vi "Autonomous Independent.vi"() -> ()   [LabVIEW 2017]
doc: "This VI is called when autonomous begins, and will automatically be terminated when autonomous ends. You can carry out timed or sensor driven robot movement independently without needing to return to the caller."
uses:
  <vilib>/Rock Robotics/WPI/ThirdParty/Sensors/navX/_TypeDefs/FRIC_navX_DeviceNumbersTypeDef.ctl
  <vilib>/Rock Robotics/WPI/Utilities/WPI_GetSetVariantRefNum.vi
  <vilib>/Rock Robotics/Network Tables/NT Read String.vi
  <vilib>/Rock Robotics/Network Tables/NT Write Numeric Array.vi
panel:
  out "error out":errorcluster
  out "Array":dbl[](array[numeric])
  out "Direction":string[](array[string])
  # "Be sure to right-click and choose Data Operations>>Make Current Value default if you want to save the array values with the VI"
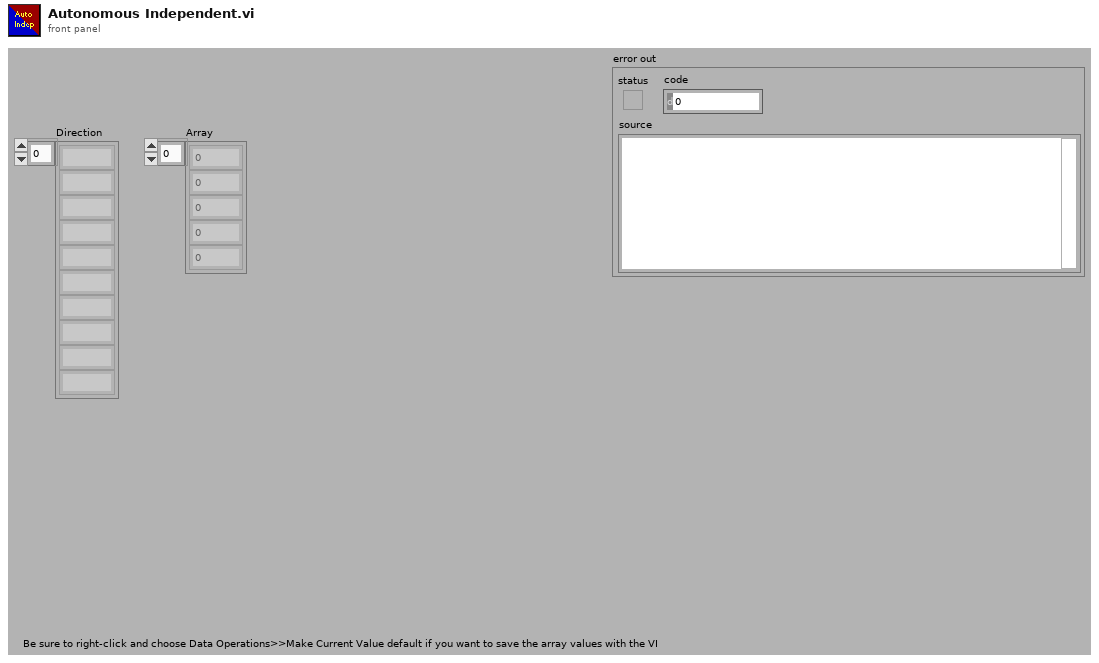
[diagram p1: front panel]
types:
  T1 = typedef "FRIC_navX_DeviceNumbersTypeDef.ctl" = enum16{"Dev0", "Dev1", "Dev2", "Dev3"}
  T2 = cluster{"Left Encoder":string, "Right Encoder":string, "Gyro Refnum":string, "Device Number":T1, "Right Refnum":string, "Left Refnum":string, "Right Intake":string, "Left Intake":string}
  T3 = typedef "WPI_JoystickDevRef.ctl" = cluster{"Device":T4}
  T4 = typedef "WPI_JoystickDeviceEnum.ctl" = enum16{"USB 0", "USB 1", "USB 2", "USB 3", "USB 4", "USB 5"}
  T5 = typedef "WPI_DriverStationPositionInfo.ctl" = enum16{"1", "2", "3"}
  T6 = cluster{"Left Encoder":string, "Right Encoder":string, "Gyro Refnum":string, "Device Number":T1, "Right Refnum":string, "Left Refnum":string, "Left Intake":string, "Right Intake":string}
  T7 = cluster{"Width":u16, "Style":enum32{"Solid", "Dash", "Dot", "DashDot", "DashDotDot"}}
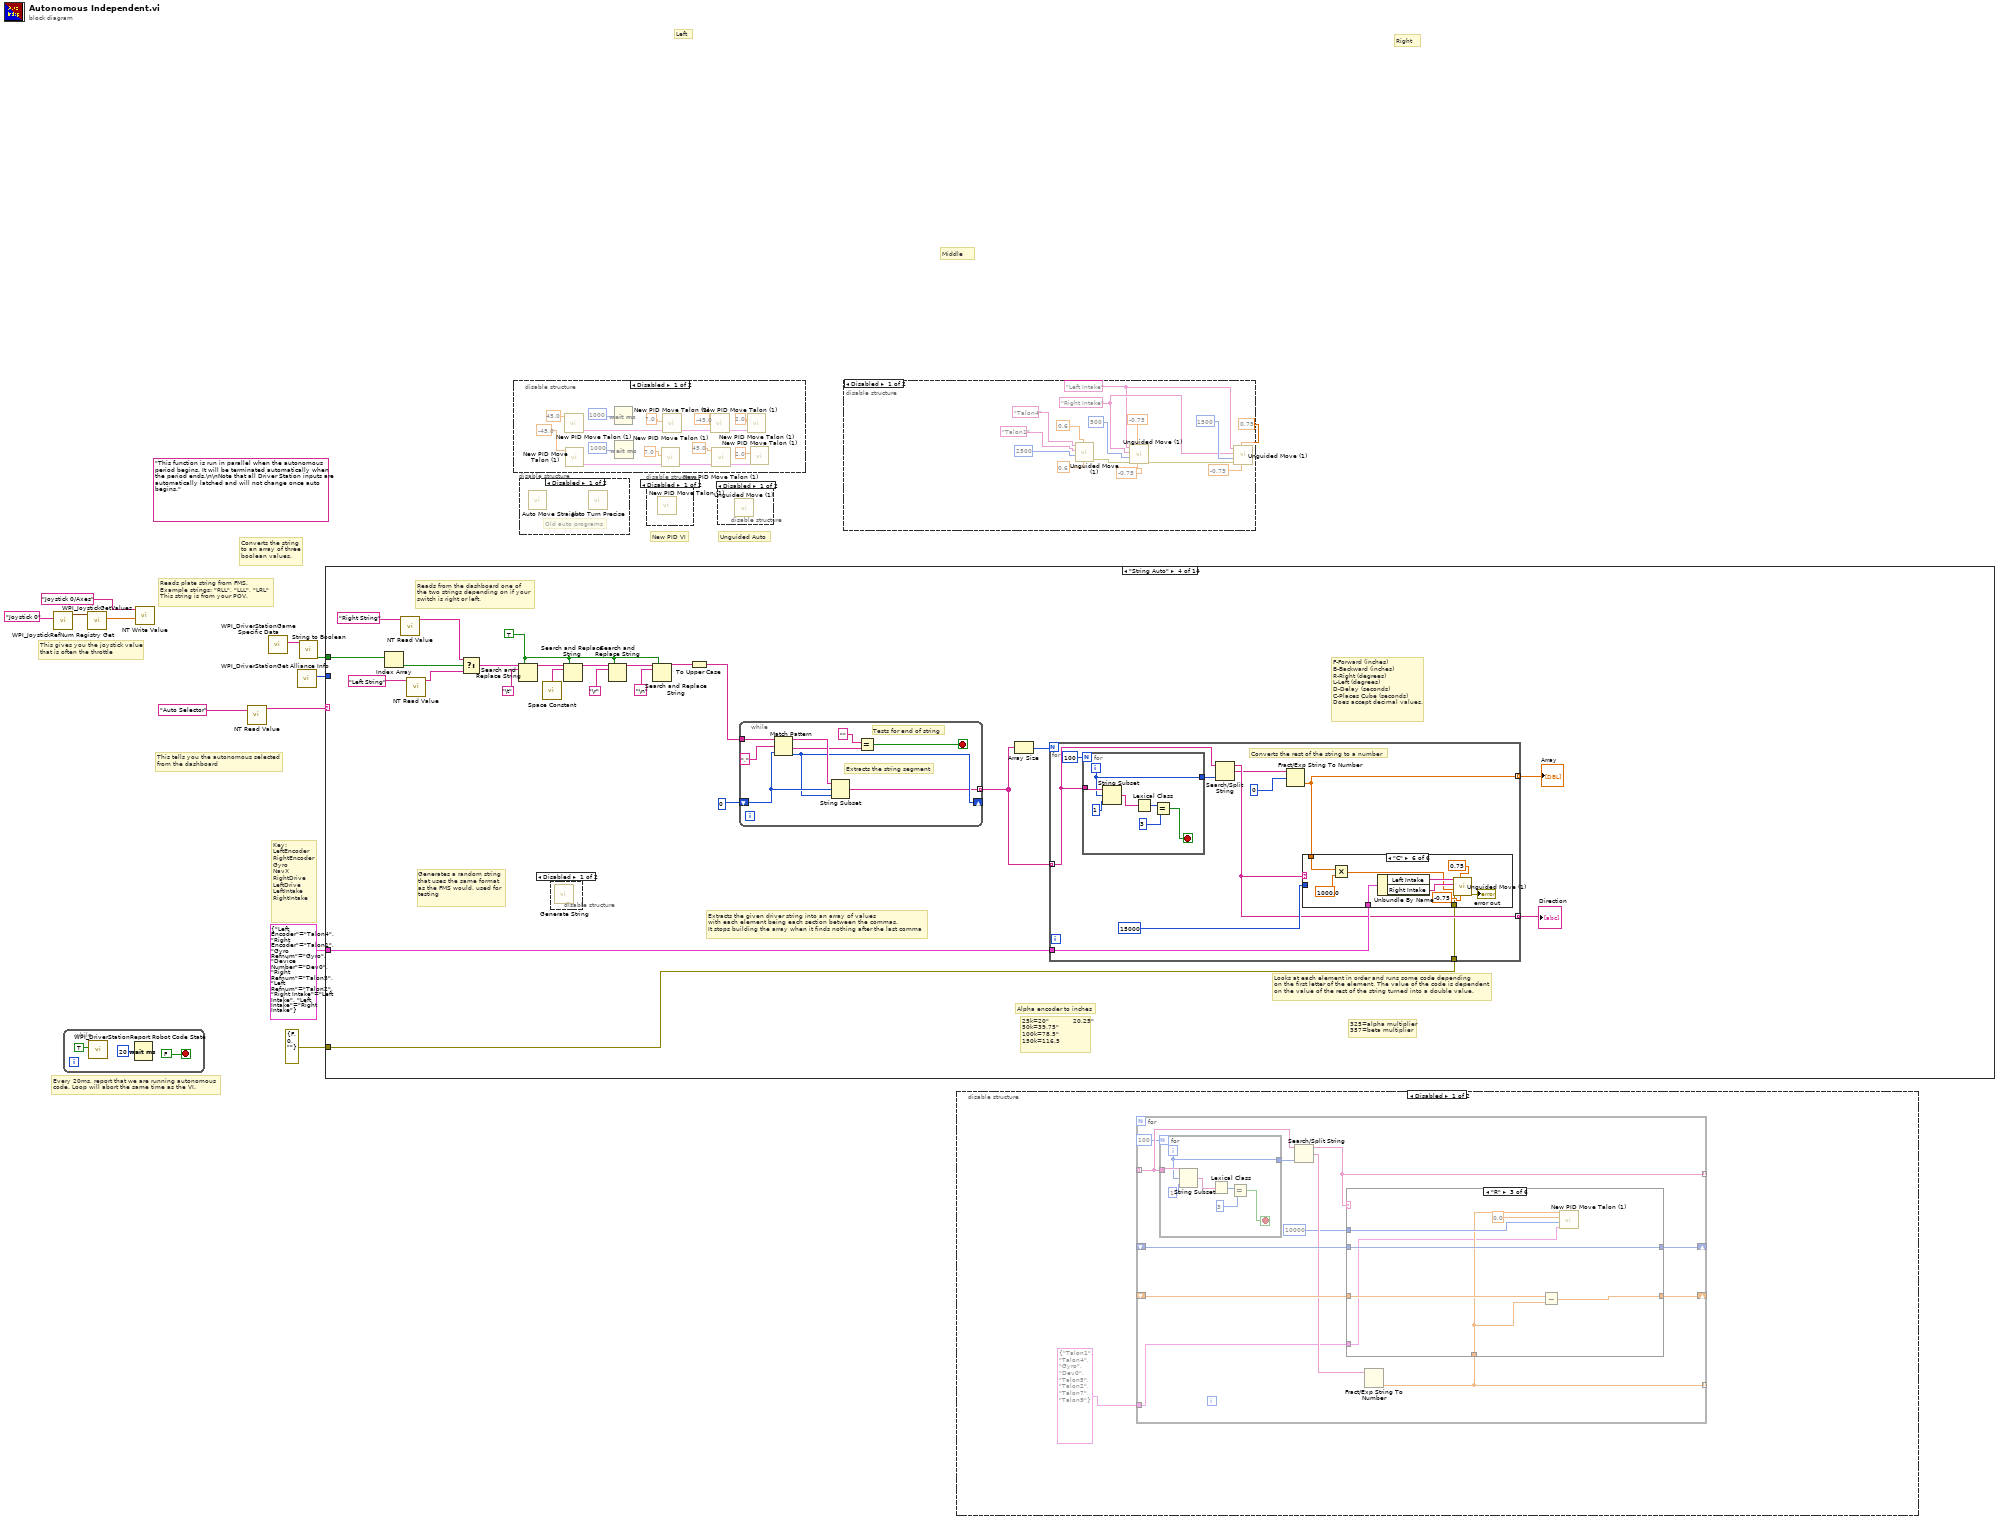
[diagram p0: block diagram]
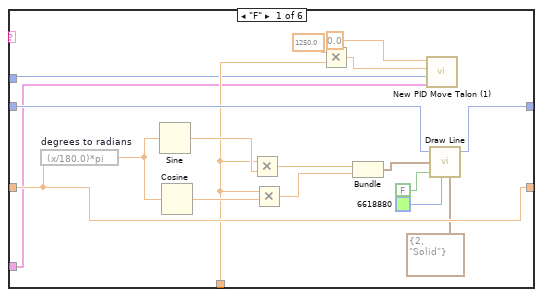
[diagram p2: hidden frame]
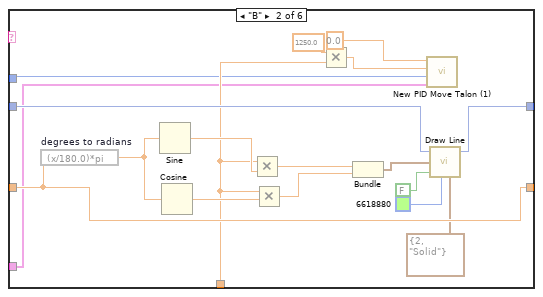
[diagram p3: hidden frame]
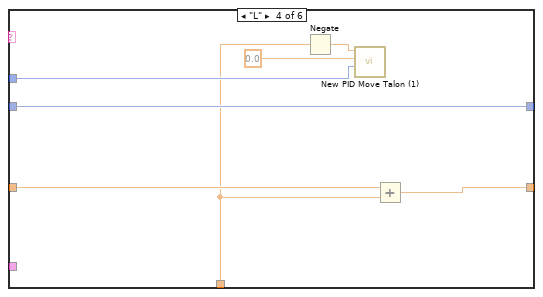
[diagram p4: hidden frame]
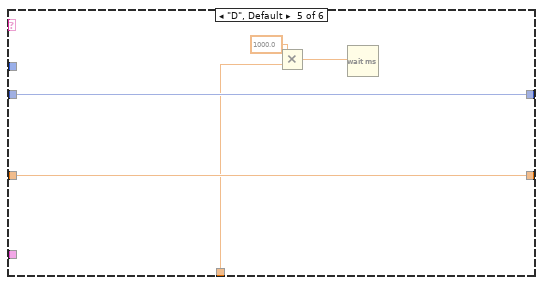
[diagram p5: hidden frame]
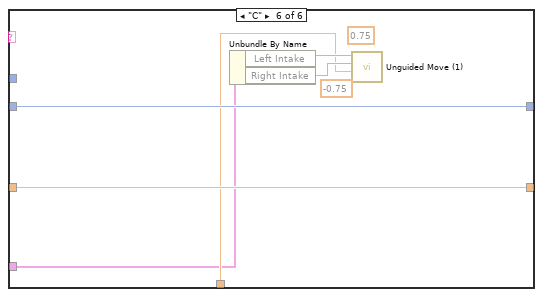
[diagram p6: hidden frame]
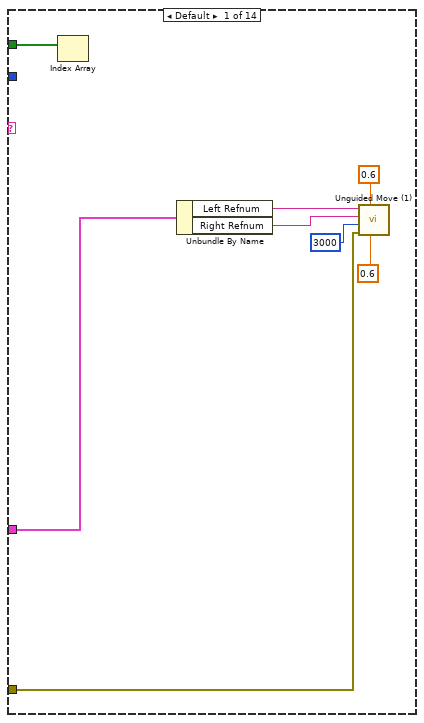
[diagram p13: hidden frame]
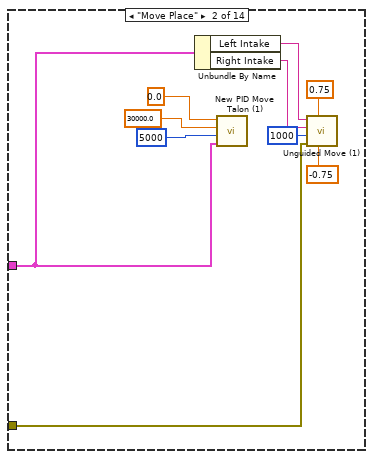
[diagram p14: hidden frame]
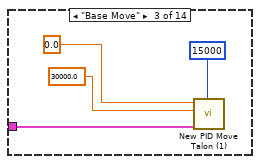
[diagram p15: hidden frame]
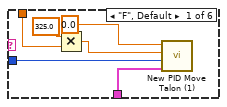
[diagram p17: hidden frame]
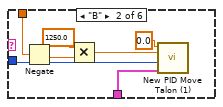
[diagram p18: hidden frame]
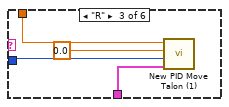
[diagram p19: hidden frame]
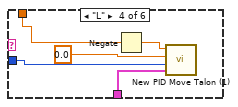
[diagram p20: hidden frame]
diagram:
  (unwired) "This function is run in parallel when the autonomous period begins. It will be terminated automatically when the period ends.\n\nNote that all Driver Station inputs are automatically latched and will not change once auto begins."
  # "Key:\nLeftEncoder\nRightEncoder\nGyro\nNavX\nRightDrive\nLeftDrive\nLeftIntake\nRightIntake"
  # "Unguided Auto"
  # "New PID VI"
  # "Converts the string\nto an array of three\nboolean values."
  # "Reads plate string from FMS. \nExample strings: \"RLL\", \"LLL\", \"LRL\"\nThis string is from your POV."
  # "Middle"
  # "Left"
  # "Right"
  # "This tells you the autonomous selected\nfrom the dashboard"
  # "Every 20ms, report that we are running autonomous\ncode. Loop will abort the same time as the VI."
  # "This gives you the joystick value\nthat is often the throttle"
  n1 = call <vilib>:"WPI_JoystickRefNum Registry Get.vi"("refnum name"="Joystick 0") -> ("JoystickDevRef"=w10:T3)  [unwired: 1 in, 9 out]
  n2 = while {
    stop <- FALSE stop-if-true
    n3 = call <vilib>:"WPI_DriverStationReport Robot Code State.vi"("Autonomous"=TRUE) -> ()  [unwired: 10 in, 1 out]
    n4 = Wait (ms)(milliseconds to wait=u32 20) -> ()  [unwired: 1 out]
  }
  n5 = call <vilib>:"WPI_JoystickGetValues.vi"("JoystickDevRef"=w10) -> ("Axes"=w7:dbl[])  [unwired: 6 in, 4 out]
  n6 = call-poly <vilib>:"NT Write Value.vi"("Numeric Array"=w7, "Name"="Joystick 0/Axes") -> ()  [unwired: 9 in, 1 out]
  n7 = call-poly <vilib>:"NT Read Value.vi"("Name"="Auto Selector") -> ("String"=w8:string)  [unwired: 9 in, 1 out]
  n8 = call <vilib>:"WPI_DriverStationGame Specific Data.vi"() -> ("Game Specific Data"=w5:string)  [unwired: 11 in]
  n9 = call <vilib>:"WPI_DriverStationGet Alliance Info.vi"() -> ("Position"=w1:T5)  [unwired: 6 in, 5 out]
  n10 = call "String to Boolean.vi"("String"=w5) -> ("Boolean Array"=w4:bool[])  [unwired: 10 in]
  n11 = case shown="\"String Auto\"" w8 {
    tunnel: w4 -> [w15 _ _ w50 w124 _ _ w172 _ _ _ _ _ _]
    tunnel: T2 {"Left Encoder"="Talon4", "Right Encoder"="Talon1", "Gyro Refnum"="Gyro", "Device Number"=enum."Dev0", "Right Refnum"="Talon5", "Left Refnum"="Talon2", "Right Intake"="Left Intake", "Left Intake"="Right Intake"} ("Cluster 3") -> [w16 w32 w33 w38 _ _ _ _ _ _ _ _ _ _]
    tunnel: errorcluster {"status"=FALSE, "code"=0, "source"=""} ("error in (no error)") -> [w19 w26 _ w37 _ _ _ _ _ _ _ _ _ _]
    tunnel: w1 -> [_ _ _ _ _ _ _ _ _ _ _ _ _ _]
    frame Default {
      n12 = Index Array(array=w15) -> ()  [unwired: 1 in, 1 out]
      n13 = Unbundle By Name(w16) -> ("Left Refnum"=w22:string, "Right Refnum"=w21:string)
      n14 = call "Unguided Move (1).vi"("Power 2"=0.6, "Power"=0.6, "error in (no error)"=w19, "milliseconds to wait"=u32 3000, "refnum name 2"=w21, "refnum name"=w22) -> ()  [unwired: 5 in, 1 out]
    }
    frame "Move Place" {
      n15 = Unbundle By Name(w32) -> ("Left Intake"=w28:string, "Right Intake"=w27:string)
      n16 = call "New PID Move Talon (1).vi"("Cluster 3"=w32, "Timeout"=i16 5000, "Target Distance"=30000.0, "Target Angle"=0.0) -> ()  [unwired: 7 in, 1 out]
      n17 = call "Unguided Move (1).vi"("Power 2"=-0.75, "Power"=0.75 ("Power 2"), "error in (no error)"=w26, "milliseconds to wait"=u32 1000, "refnum name 2"=w27, "refnum name"=w28) -> ()  [unwired: 5 in, 1 out]
    }
    frame "Base Move" {
      n18 = call "New PID Move Talon (1).vi"("Cluster 3"=w33, "Timeout"=i16 15000, "Target Distance"=30000.0, "Target Angle"=0.0) -> ()  [unwired: 7 in, 1 out]
    }
    frame "String Auto" {
      w42 = TRUE ("replace all? (F)")
      # "325=alpha multiplier\n357=beta multiplier"
      # "F-Forward (inches)\nB-Backward (inches)\nR-Right (degrees)\nL-Left (degrees)\nD-Delay (seconds)\nC-Places Cube (seconds)\nDoes accept decimal values."
      # "Alpha encoder to inches"
      # "25k=20\"            20.25\"\n50k=39.75\"\n100k=78.5\"\n150k=116.5"
      # "Looks at each element in order and runs some code depending\non the first letter of the element. The value of the code is dependent\non the value of the rest of the string turned into a double value."
      # "Extracts the given driver string into an array of values \nwith each element being each section between the commas.\nIt stops building the array when it finds nothing after the last comma"
      # "Reads from the dashboard one of\nthe two strings depending on if your\nswitch is right or left."
      # "Generates a random string\nthat uses the same format \nas the FMS would, used for\ntesting"
      n19 = Index Array(array=w50) -> (element=w60:bool)  [unwired: 1 in]
      n20 = call-poly <vilib>:"NT Read Value.vi"("Name"="Right String") -> ("String"=w59:string)  [unwired: 9 in, 1 out]
      n21 = call-poly <vilib>:"NT Read Value.vi"("Name"="Left String") -> ("String"=w56:string)  [unwired: 9 in, 1 out]
      n22 = Select(t=w59, s=w60, f=w56) -> (s? t:f=w40:string)
      n23 = Search and Replace String(replace all?=w42, input string=w40, search string="\t") -> (result string=w46:string)  [unwired: 5 in, 3 out]
      n24 = call <vilib>:"Space Constant.vi"() -> ("String"=w44:string)
      n25 = disable-structure shown="Disabled" {
        frame Disabled {
          n26 = call "Generate String.vi"() -> ()  [unwired: 11 in, 1 out]
        }
        frame Enabled {
        }
      }
      n27 = Search and Replace String(replace all?=w42, input string=w46, search string=w44) -> (result string=w47:string)  [unwired: 5 in, 3 out]
      n28 = Search and Replace String(replace all?=w42, input string=w47, search string="\r") -> (result string=w48:string)  [unwired: 5 in, 3 out]
      n29 = Search and Replace String(replace all?=w42, input string=w48, search string="\n") -> (result string=w41:string)  [unwired: 5 in, 3 out]
      n30 = To Upper Case(1:w41) -> (0:w39:string)
      n31 = while {
        tunnel: w39 -> [w121]
        shift-right: [w117] -> _
        shift-left: 0 ("offset past match") -> [w118]
        tunnel: [w116] -> w53 mode=indexing
        stop <- w113 stop-if-true
        # "Tests for end of string"
        # "Extracts the string segment"
        n32 = Match Pattern(string=w121, regular expression=",", offset (0)=w118) -> (before substring=w119:string, after substring=w115:string, offset past match=w117:i32)  [unwired: 1 out]
        n33 = String Subset(string=w119, offset (0)=w118, length (rest)=w117) -> (substring=w116:string)
        n34 = Equal?(x="", y=w115) -> (x = y?=w113:bool)
      }
      n35 = Array Size(array=w53) -> (size(s)=w54:i32)
      n36 = for {
        N: w54 -> [_]
        tunnel: w53 -> [w65] mode=indexing
        tunnel: [w69] -> w51 mode=indexing
        tunnel: [w64] -> w52 mode=indexing
        tunnel: w38 -> [w68]
        tunnel: w37 -> [w61]
        # "Converts the rest of the string to a number"
        n37 = for {
          N: 100 -> [_]
          tunnel: w65 -> [w75]
          tunnel: [w72] -> w66
          i -> [w72]
          stop <- w71 stop-if-true
          n38 = String Subset(string=w75, offset (0)=w72, length (rest)=1 ("length (rest)")) -> (substring=w73:string)
          n39 = Lexical Class(1:w73) -> (0:w77:i16)
          n40 = Equal?(x=w77, y=i16 3) -> (x = y?=w71:bool)
        }
        n41 = Search/Split String(string=w65, offset (0)=w66) -> (substring before match=w64:string, match + rest of string=w63:string)  [unwired: 1 in, 1 out]
        n42 = Fract/Exp String To Number(string=w63, offset=0) -> (number=w69:dbl)  [unwired: 2 in, 1 out]
        n43 = case shown="\"C\"" w64 {
          tunnel: w69 -> [w79 w87 w94 w97 w101 w111]
          tunnel: w68 -> [w83 w90 w92 w96 _ w112]
          tunnel: i16 15000 ("Timeout") -> [w82 w89 w91 w95 _ _]
          tunnel: w61 -> [_ _ _ _ _ w103]
          frame "F", Default {
            n44 = Multiply(x=325.0, y=w79) -> (x*y=w78:dbl)
            n45 = call "New PID Move Talon (1).vi"("Cluster 3"=w83, "Timeout"=w82, "Target Distance"=w78, "Target Angle"=0.0) -> ()  [unwired: 7 in, 1 out]
          }
          frame "B" {
            n46 = Negate(x=w87) -> (-x=w86:dbl)
            n47 = Multiply(x=1250.0, y=w86) -> (x*y=w85:dbl)
            n48 = call "New PID Move Talon (1).vi"("Cluster 3"=w90, "Timeout"=w89, "Target Distance"=w85, "Target Angle"=0.0) -> ()  [unwired: 7 in, 1 out]
          }
          frame "R" {
            n49 = call "New PID Move Talon (1).vi"("Cluster 3"=w92, "Timeout"=w91, "Target Distance"=0.0, "Target Angle"=w94) -> ()  [unwired: 7 in, 1 out]
          }
          frame "L" {
            n50 = Negate(x=w97) -> (-x=w98:dbl)
            n51 = call "New PID Move Talon (1).vi"("Cluster 3"=w96, "Timeout"=w95, "Target Distance"=0.0, "Target Angle"=w98) -> ()  [unwired: 7 in, 1 out]
          }
          frame "D" {
            n52 = Multiply(x=1000.0, y=w101) -> (x*y=w100:dbl)
            n53 = Wait (ms)(milliseconds to wait=w100) -> ()  [unwired: 1 out]
          }
          frame "C" {
            n54 = Multiply(x=w111, y=1000.0) -> (x*y=w107:dbl)
            n55 = Unbundle By Name(w112) -> ("Left Intake"=w108:string, "Right Intake"=w109:string)
            n56 = call "Unguided Move (1).vi"("Power 2"=-0.75, "Power"=0.75, "error in (no error)"=w103, "milliseconds to wait"=w107, "refnum name 2"=w109, "refnum name"=w108) -> ("error out"=→"error out":errorcluster)  [unwired: 5 in]
          }
        }
      }
      "Direction" <- w52
      "Array" <- w51
    }
    frame "Front Left Auto" {
      w127 = "Right Intake" ("refnum name")
      w125 = "Left Intake" ("refnum name")
      n57 = Index Array(array=w124) -> (element=w123:bool)  [unwired: 1 in]
      n58 = Not(x=w123) -> (.not. x?=w122:bool)
      n59 = call "Unguided Move (1).vi"("Power 2"=0.6, "Power"=0.6, "milliseconds to wait"=u32 2500, "refnum name 2"="Talon1", "refnum name"="Talon4") -> ("error out"=w129:errorcluster)  [unwired: 6 in]
      n60 = call "Unguided Move (1).vi"("Power 2"=-0.75 ("Power"), "Power"=-0.75, "error in (no error)"=w129, "milliseconds to wait"=u32 500, "refnum name 2"=w127, "refnum name"=w125) -> ("error out"=w126:errorcluster)  [unwired: 5 in]
      n61 = case shown="True" w122 {
        tunnel: w127 -> [_ w142]
        tunnel: w126 -> [_ w139]
        tunnel: w125 -> [_ w138]
        frame False {
        }
        frame True {
          n62 = call "Unguided Move (1).vi"("Power 2"=-0.75, "Power"=0.75, "error in (no error)"=w139, "milliseconds to wait"=u32 1500, "refnum name 2"=w142, "refnum name"=w138) -> ()  [unwired: 5 in, 1 out]
        }
      }
      n63 = disable-structure shown="Enabled" {
        frame Disabled {
          n64 = call "New PID Move Talon (1).vi"("Target Distance"=4.0 ("Target Angle")) -> ("Cluster 2"=w149:T2)  [unwired: 10 in]
          n65 = call "New PID Move Talon (1).vi"("Cluster 3"=w149, "Target Angle"=90.0 ("Target Distance")) -> ("Cluster 2"=w150:T2)  [unwired: 9 in]
          n66 = call "New PID Move Talon (1).vi"("Cluster 3"=w150, "Target Distance"=5.0 ("Target Angle")) -> ("Cluster 2"=w148:T2)  [unwired: 9 in]
          n67 = call "New PID Move Talon (1).vi"("Cluster 3"=w148, "Target Angle"=-90.0 ("Target Distance")) -> ("Cluster 2"=w151:T2)  [unwired: 9 in]
          n68 = call "New PID Move Talon (1).vi"("Cluster 3"=w151, "Target Distance"=5.0) -> ()  [unwired: 9 in, 1 out]
        }
        frame Enabled {
        }
      }
    }
    frame "Side Left Auto" {
      w152 = i16 15000 ("Timeout")
      n69 = call "New PID Move Talon (1).vi"("Timeout"=w152, "Target Distance"=150000.0) -> ("Cluster 2"=w157:T2)  [unwired: 9 in]
      n70 = call "New PID Move Talon (1).vi"("Cluster 3"=w157, "Timeout"=w152, "Target Angle"=90.0) -> ("Cluster 2"=w156:T2)  [unwired: 8 in]
      n71 = call "New PID Move Talon (1).vi"("Cluster 3"=w156, "Timeout"=w152, "Target Distance"=10000.0) -> ()  [unwired: 8 in, 1 out]
    }
    frame "Other Side Left Auto" {
      n72 = call "New PID Move Talon (1).vi"("Target Distance"=18.5 ("Target Angle")) -> ("Cluster 2"=w166:T2)  [unwired: 10 in]
      n73 = call "New PID Move Talon (1).vi"("Cluster 3"=w166, "Target Angle"=90.0 ("Target Distance")) -> ("Cluster 2"=w167:T2)  [unwired: 9 in]
      n74 = call "New PID Move Talon (1).vi"("Cluster 3"=w167, "Target Distance"=18.0 ("Target Angle")) -> ("Cluster 2"=w165:T2)  [unwired: 9 in]
      n75 = call "New PID Move Talon (1).vi"("Cluster 3"=w165, "Target Angle"=90.0 ("Target Distance")) -> ("Cluster 2"=w168:T2)  [unwired: 9 in]
      n76 = call "New PID Move Talon (1).vi"("Cluster 3"=w168, "Target Distance"=5.0) -> ("Cluster 2"=w169:T2)  [unwired: 9 in]
      n77 = call "New PID Move Talon (1).vi"("Cluster 3"=w169, "Target Angle"=90.0) -> ("Cluster 2"=w170:T2)  [unwired: 9 in]
      n78 = call "New PID Move Talon (1).vi"("Cluster 3"=w170, "Target Distance"=1.0) -> ()  [unwired: 9 in, 1 out]
    }
    frame "Front Right Auto" {
      w175 = "Right Intake" ("refnum name")
      w173 = "Left Intake" ("refnum name")
      n79 = Index Array(array=w172) -> (element=w171:bool)  [unwired: 1 in]
      n80 = call "Unguided Move (1).vi"("Power 2"=0.6, "Power"=0.6, "milliseconds to wait"=u32 2500, "refnum name 2"="Talon2", "refnum name"="Talon5") -> ("error out"=w177:errorcluster)  [unwired: 6 in]
      n81 = call "Unguided Move (1).vi"("Power 2"=-0.75 ("Power"), "Power"=-0.75, "error in (no error)"=w177, "milliseconds to wait"=u32 500, "refnum name 2"=w175, "refnum name"=w173) -> ("error out"=w174:errorcluster)  [unwired: 5 in]
      n82 = case shown="True" w171 {
        tunnel: w175 -> [_ w190]
        tunnel: w174 -> [_ w187]
        tunnel: w173 -> [_ w186]
        frame False {
        }
        frame True {
          n83 = call "Unguided Move (1).vi"("Power 2"=-0.75, "Power"=0.75, "error in (no error)"=w187, "milliseconds to wait"=u32 1500, "refnum name 2"=w190, "refnum name"=w186) -> ()  [unwired: 5 in, 1 out]
        }
      }
      n84 = disable-structure shown="Disabled" {
        frame Disabled {
          n85 = call "New PID Move Talon (1).vi"("Target Distance"=4.0 ("Target Angle")) -> ("Cluster 2"=w197:T2)  [unwired: 10 in]
          n86 = call "New PID Move Talon (1).vi"("Cluster 3"=w197, "Target Angle"=-90.0 ("Target Distance")) -> ("Cluster 2"=w198:T2)  [unwired: 9 in]
          n87 = call "New PID Move Talon (1).vi"("Cluster 3"=w198, "Target Distance"=5.0 ("Target Angle")) -> ("Cluster 2"=w196:T2)  [unwired: 9 in]
          n88 = call "New PID Move Talon (1).vi"("Cluster 3"=w196, "Target Angle"=90.0 ("Target Distance")) -> ("Cluster 2"=w199:T2)  [unwired: 9 in]
          n89 = call "New PID Move Talon (1).vi"("Cluster 3"=w199, "Target Distance"=5.0) -> ()  [unwired: 9 in, 1 out]
        }
        frame Enabled {
        }
      }
    }
    frame "Side Right Auto" {
      n90 = call "New PID Move Talon (1).vi"("Target Distance"=12.0) -> ("Cluster 2"=w204:T2)  [unwired: 10 in]
      n91 = call "New PID Move Talon (1).vi"("Cluster 3"=w204, "Target Angle"=-90.0) -> ("Cluster 2"=w203:T2)  [unwired: 9 in]
      n92 = call "New PID Move Talon (1).vi"("Cluster 3"=w203, "Target Distance"=1.5) -> ()  [unwired: 9 in, 1 out]
    }
    frame "Other Side Right Auto" {
      n93 = call "New PID Move Talon (1).vi"("Target Distance"=18.5 ("Target Angle")) -> ("Cluster 2"=w213:T2)  [unwired: 10 in]
      n94 = call "New PID Move Talon (1).vi"("Cluster 3"=w213, "Target Angle"=-90.0 ("Target Distance")) -> ("Cluster 2"=w214:T2)  [unwired: 9 in]
      n95 = call "New PID Move Talon (1).vi"("Cluster 3"=w214, "Target Distance"=18.0 ("Target Angle")) -> ("Cluster 2"=w212:T2)  [unwired: 9 in]
      n96 = call "New PID Move Talon (1).vi"("Cluster 3"=w212, "Target Angle"=-90.0 ("Target Distance")) -> ("Cluster 2"=w215:T2)  [unwired: 9 in]
      n97 = call "New PID Move Talon (1).vi"("Cluster 3"=w215, "Target Distance"=5.0) -> ("Cluster 2"=w216:T2)  [unwired: 9 in]
      n98 = call "New PID Move Talon (1).vi"("Cluster 3"=w216, "Target Angle"=-90.0) -> ("Cluster 2"=w217:T2)  [unwired: 9 in]
      n99 = call "New PID Move Talon (1).vi"("Cluster 3"=w217, "Target Distance"=1.0) -> ()  [unwired: 9 in, 1 out]
    }
    frame "Middle Left Side Auto" {
      n100 = call "New PID Move Talon (1).vi"("Target Distance"=5.0) -> ("Cluster 2"=w224:T2)  [unwired: 10 in]
      n101 = call "New PID Move Talon (1).vi"("Cluster 3"=w224, "Target Angle"=-90.0) -> ("Cluster 2"=w225:T2)  [unwired: 9 in]
      n102 = call "New PID Move Talon (1).vi"("Cluster 3"=w225, "Target Distance"=13.0) -> ("Cluster 2"=w226:T2)  [unwired: 9 in]
      n103 = call "New PID Move Talon (1).vi"("Cluster 3"=w226, "Target Distance"=7.0 ("Target Angle")) -> ("Cluster 2"=w227:T2)  [unwired: 9 in]
      n104 = call "New PID Move Talon (1).vi"("Cluster 3"=w227, "Target Angle"=90.0 ("Target Distance")) -> ("Cluster 2"=w228:T2)  [unwired: 9 in]
      n105 = call "New PID Move Talon (1).vi"("Cluster 3"=w228, "Target Distance"=1.0) -> ()  [unwired: 9 in, 1 out]
    }
    frame "Middle Right Front Auto" {
      n106 = call "New PID Move Talon (1).vi"("Target Distance"=9.0) -> ()  [unwired: 10 in, 1 out]
    }
    frame "Middle Right Side Auto" {
      n107 = call "New PID Move Talon (1).vi"("Target Distance"=6.0) -> ("Cluster 2"=w237:T2)  [unwired: 10 in]
      n108 = call "New PID Move Talon (1).vi"("Cluster 3"=w237, "Target Angle"=90.0) -> ("Cluster 2"=w238:T2)  [unwired: 9 in]
      n109 = call "New PID Move Talon (1).vi"("Cluster 3"=w238, "Target Distance"=4.0) -> ("Cluster 2"=w239:T2)  [unwired: 9 in]
      n110 = call "New PID Move Talon (1).vi"("Cluster 3"=w239, "Target Angle"=-90.0) -> ("Cluster 2"=w240:T2)  [unwired: 9 in]
      n111 = call "New PID Move Talon (1).vi"("Cluster 3"=w240, "Target Distance"=7.0) -> ("Cluster 2"=w241:T2)  [unwired: 9 in]
      n112 = call "New PID Move Talon (1).vi"("Cluster 3"=w241, "Target Angle"=-90.0) -> ("Cluster 2"=w242:T2)  [unwired: 9 in]
      n113 = call "New PID Move Talon (1).vi"("Cluster 3"=w242, "Target Distance"=1.0) -> ()  [unwired: 9 in, 1 out]
    }
    frame "Middle Left Front Auto" {
      n114 = call "New PID Move Talon (1).vi"("Target Distance"=4.0) -> ("Cluster 2"=w248:T2)  [unwired: 10 in]
      n115 = call "New PID Move Talon (1).vi"("Cluster 3"=w248, "Target Angle"=-90.0) -> ("Cluster 2"=w249:T2)  [unwired: 9 in]
      n116 = call "New PID Move Talon (1).vi"("Cluster 3"=w249, "Target Distance"=9.0) -> ("Cluster 2"=w250:T2)  [unwired: 9 in]
      n117 = call "New PID Move Talon (1).vi"("Cluster 3"=w250, "Target Angle"=90.0) -> ("Cluster 2"=w251:T2)  [unwired: 9 in]
      n118 = call "New PID Move Talon (1).vi"("Cluster 3"=w251, "Target Distance"=5.0) -> ()  [unwired: 9 in, 1 out]
    }
  }
  n119 = disable-structure shown="Disabled" {
    frame Disabled {
      n120 = call "New PID Move Talon (1).vi"("Target Angle"=45.0) -> ("Cluster 2"=w262:T2)  [unwired: 10 in]
      n121 = call "New PID Move Talon (1).vi"("Target Angle"=-45.0) -> ("Cluster 2"=w255:T2)  [unwired: 10 in]
      n122 = Wait (ms)(milliseconds to wait=u32 1000) -> ()  [unwired: 1 out]
      n123 = Wait (ms)(milliseconds to wait=u32 1000) -> ()  [unwired: 1 out]
      n124 = call "New PID Move Talon (1).vi"("Cluster 3"=w255, "Target Distance"=7.0) -> ("Cluster 2"=w254:T2)  [unwired: 9 in]
      n125 = call "New PID Move Talon (1).vi"("Cluster 3"=w262, "Target Distance"=7.0) -> ("Cluster 2"=w261:T2)  [unwired: 9 in]
      n126 = call "New PID Move Talon (1).vi"("Cluster 3"=w261, "Target Angle"=-45.0) -> ("Cluster 2"=w260:T2)  [unwired: 9 in]
      n127 = call "New PID Move Talon (1).vi"("Cluster 3"=w254, "Target Angle"=45.0) -> ("Cluster 2"=w253:T2)  [unwired: 9 in]
      n128 = call "New PID Move Talon (1).vi"("Cluster 3"=w260, "Target Distance"=2.0) -> ()  [unwired: 9 in, 1 out]
      n129 = call "New PID Move Talon (1).vi"("Cluster 3"=w253, "Target Distance"=2.0) -> ()  [unwired: 9 in, 1 out]
    }
    frame Enabled {
    }
  }
  n130 = disable-structure shown="Disabled" {
    frame Disabled {
      # "Old auto programs"
      n131 = call "Auto Move Straight.vi"() -> ()  [unwired: 10 in, 2 out]
      n132 = call "Auto Turn Precise.vi"() -> ()  [unwired: 10 in, 2 out]
    }
    frame Enabled {
    }
  }
  n133 = disable-structure shown="Disabled" {
    frame Disabled {
      n134 = call "New PID Move Talon (1).vi"() -> ()  [unwired: 11 in, 1 out]
    }
    frame Enabled {
    }
  }
  n135 = disable-structure shown="Disabled" {
    frame Disabled {
      n136 = call "Unguided Move (1).vi"() -> ()  [unwired: 11 in, 1 out]
    }
    frame Enabled {
    }
  }
  n137 = disable-structure shown="Disabled" {
    frame Disabled {
      w278 = "Right Intake" ("refnum name")
      w277 = "Left Intake" ("refnum name")
      n138 = call "Unguided Move (1).vi"("Power 2"=0.6, "Power"=0.6, "milliseconds to wait"=u32 2500, "refnum name 2"="Talon1", "refnum name"="Talon4") -> ("error out"=w275:errorcluster)  [unwired: 6 in]
      n139 = call "Unguided Move (1).vi"("Power 2"=-0.75 ("Power"), "Power"=-0.75, "error in (no error)"=w275, "milliseconds to wait"=u32 500, "refnum name 2"=w278, "refnum name"=w277) -> ("error out"=w282:errorcluster)  [unwired: 5 in]
      n140 = call "Unguided Move (1).vi"("Power 2"=-0.75, "Power"=0.75, "error in (no error)"=w282, "milliseconds to wait"=u32 1500, "refnum name 2"=w278, "refnum name"=w277) -> ()  [unwired: 5 in, 1 out]
    }
    frame Enabled {
    }
  }
  n141 = disable-structure shown="Disabled" {
    frame Disabled {
      n142 = for {
        tunnel: [w295] -> _ mode=indexing
        tunnel: [w288] -> _ mode=indexing
        tunnel: _ -> [w289] mode=indexing
        shift-right: [w293] -> _
        shift-left: _ -> [w294]
        shift-right: [w291] -> _
        shift-left: _ -> [w292]
        tunnel: T6 {"Left Encoder"="Talon1", "Right Encoder"="Talon4", "Gyro Refnum"="Gyro", "Device Number"=enum."Dev0", "Right Refnum"="Talon5", "Left Refnum"="Talon2", "Left Intake"="Talon7", "Right Intake"="Talon9"} ("Cluster 3") -> [w284]
        n143 = for {
          N: 100 -> [_]
          tunnel: w289 -> [w361]
          tunnel: [w358] -> w290
          i -> [w358]
          stop <- w357 stop-if-true
          n144 = String Subset(string=w361, offset (0)=w358, length (rest)=1 ("length (rest)")) -> (substring=w359:string)
          n145 = Lexical Class(1:w359) -> (0:w363:i16)
          n146 = Equal?(x=w363, y=i16 3) -> (x = y?=w357:bool)
        }
        n147 = Search/Split String(string=w289, offset (0)=w290) -> (substring before match=w288:string, match + rest of string=w287:string)  [unwired: 1 in, 1 out]
        n148 = Fract/Exp String To Number(string=w287) -> (number=w295:dbl)  [unwired: 3 in, 1 out]
        n149 = case shown="\"R\"" w288 {
          tunnel: w295 -> [w298 w316 w333 w339 w346 w352]
          tunnel: w294 -> [w312 w330 w338 w345 w350 w356]
          tunnel: [w311 w329 w338 w345 w350 w356] -> w293
          tunnel: w292 -> [w305 w323 w336 w343 w349 w355]
          tunnel: [w305 w323 w337 w344 w349 w355] -> w291
          tunnel: i16 10000 ("Timeout") -> [w297 w315 w334 w340 _ _]
          tunnel: w284 -> [w296 w314 w332 _ _ w351]
          frame "F" {
            n150 = expression code="(x/180.0)*pi" "degrees to radians"(w305) -> (w308:dbl)
            n151 = Sine(x=w308) -> (sin(x)=w306:dbl)
            n152 = Cosine(x=w308) -> (cos(x)=w307:dbl)
            n153 = Multiply(x=w298, y=w306) -> (x*y=w310:dbl)
            n154 = Multiply(x=w298, y=w307) -> (x*y=w309:dbl)
            n155 = Multiply(x=1250.0, y=w298) -> (x*y=w301:dbl)
            n156 = Bundle(w310, w309) -> (w302:cluster{dbl, dbl})  [unwired: 1 in]
            n157 = call "New PID Move Talon (1).vi"("Cluster 3"=w296, "Timeout"=w297, "Target Distance"=w301, "Target Angle"=0.0) -> ()  [unwired: 7 in, 1 out]
            n158 = call <vilib>:"Draw Line.vi"("picture"=w312, "end point"=w302, "absolute coordinates?(T)"=FALSE, "color(black)"=u32 6618880, "pen"=T7 {"Width"=2, "Style"=enum."Solid"}) -> ("new picture"=w311:picture)  [unwired: 4 in]
          }
          frame "B" {
            n159 = expression code="(x/180.0)*pi" "degrees to radians"(w323) -> (w326:dbl)
            n160 = Sine(x=w326) -> (sin(x)=w324:dbl)
            n161 = Cosine(x=w326) -> (cos(x)=w325:dbl)
            n162 = Multiply(x=w316, y=w324) -> (x*y=w328:dbl)
            n163 = Multiply(x=w316, y=w325) -> (x*y=w327:dbl)
            n164 = Multiply(x=1250.0, y=w316) -> (x*y=w319:dbl)
            n165 = Bundle(w328, w327) -> (w320:cluster{dbl, dbl})  [unwired: 1 in]
            n166 = call "New PID Move Talon (1).vi"("Cluster 3"=w314, "Timeout"=w315, "Target Distance"=w319, "Target Angle"=0.0) -> ()  [unwired: 7 in, 1 out]
            n167 = call <vilib>:"Draw Line.vi"("picture"=w330, "end point"=w320, "absolute coordinates?(T)"=FALSE, "color(black)"=u32 6618880, "pen"=T7 {"Width"=2, "Style"=enum."Solid"}) -> ("new picture"=w329:picture)  [unwired: 4 in]
          }
          frame "R" {
            n168 = Subtract(x=w336, y=w333) -> (x-y=w337:dbl)
            n169 = call "New PID Move Talon (1).vi"("Cluster 3"=w332, "Timeout"=w334, "Target Distance"=0.0, "Target Angle"=w333) -> ()  [unwired: 7 in, 1 out]
          }
          frame "L" {
            n170 = Negate(x=w339) -> (-x=w342:dbl)
            n171 = call "New PID Move Talon (1).vi"("Timeout"=w340, "Target Distance"=0.0, "Target Angle"=w342) -> ()  [unwired: 8 in, 1 out]
            n172 = Add(x=w343, y=w339) -> (x+y=w344:dbl)
          }
          frame "D", Default {
            n173 = Multiply(x=1000.0, y=w346) -> (x*y=w348:dbl)
            n174 = Wait (ms)(milliseconds to wait=w348) -> ()  [unwired: 1 out]
          }
          frame "C" {
            (unwired) -0.75 ("Power 2")
            (unwired) 0.75 ("Power")
            n175 = Unbundle By Name(w351) -> ("Left Intake"=w354:string, "Right Intake"=w353:string)
            n176 = call "Unguided Move (1).vi"("milliseconds to wait"=w352, "refnum name 2"=w353, "refnum name"=w354) -> ()  [unwired: 8 in, 1 out]
          }
        }
      }
    }
    frame Enabled {
    }
  }
